vi "r_db_create.vi"(6 "ms timeout (0:default)":i32, 7 "db":string, 8 "error in (no error)":errorcluster, 11 "rethinkdb in":T1) -> (0 "error out":errorcluster, 1 "response":variant, 2 "db exists?":bool, 3 "rethinkdb out":T1)   [LabVIEW 2017, in "rethinkdb.lvlib"]
uses:
  rethinkdb.lvlib
  refnum.ctl
  ql2_term.ctl
  ql2_query.ctl
  ql2_term_to_id.vi
  ql2_query_to_id.vi
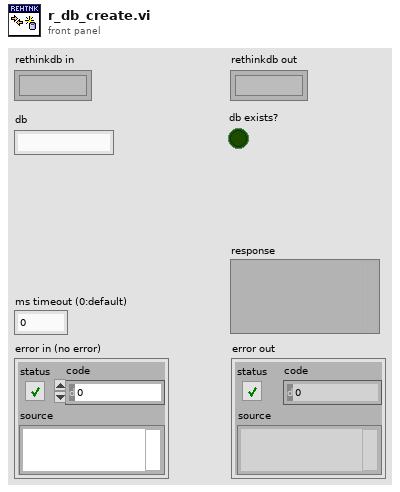
[diagram p1: front panel]
types:
  T1 = typedef "rethinkdb.lvlib/refnum.ctl" = refnum<k1>
  T2 = typedef "rethinkdb.lvlib/ql2_query.ctl" = enum8{"START", "CONTINUE", "STOP", "NOREPLY_WAIT", "SERVER_INFO", "invalid"}
  T3 = typedef "rethinkdb.lvlib/ql2_term.ctl" = enum8{"ADD", "AND", "APPEND", "APRIL", "ARGS", "ASC", "AUGUST", "AVG", "BETWEEN", "BETWEEN_DEPRECATED", "BINARY", "BIT_AND", "BIT_NOT", "BIT_OR", "BIT_SAL", "BIT_SAR", "BIT_XOR", "BRACKET", "BRANCH", "CEIL", "CHANGES", "CHANGE_AT", "CIRCLE", "COERCE_TO", "CONCAT_MAP", "CONFIG", "CONTAINS", "COUNT", "DATE", "DATUM", "DAY", "DAY_OF_WEEK", "DAY_OF_YEAR", "DB", "DB_CREATE", "DB_DROP", "DB_LIST", "DECEMBER", "DEFAULT", "DELETE", "DELETE_AT", "DESC", "DIFFERENCE", "DISTANCE", "DISTINCT", "DIV", "DOWNCASE", "DURING", "EPOCH_TIME", "EQ", "EQ_JOIN", "ERROR", "FEBRUARY", "FILL", "FILTER", "FLOOR", "FOLD", "FOR_EACH", "FRIDAY", "FUNC", "FUNCALL", "GE", "GEOJSON", "GET", "GET_ALL", "GET_FIELD", "GET_INTERSECTING", "GET_NEAREST", "GET_WRITE_HOOK", "GRANT", "GROUP", "GT", "HAS_FIELDS", "HOURS", "HTTP", "IMPLICIT_VAR", "INCLUDES", "INDEX_CREATE", "INDEX_DROP", "INDEX_LIST", "INDEX_RENAME", "INDEX_STATUS", "INDEX_WAIT", "INFO", "INNER_JOIN", "INSERT", "INSERT_AT", "INTERSECTS", "IN_TIMEZONE", "ISO8601", "IS_EMPTY", "JANUARY", "JAVASCRIPT", "JSON", "JULY", "JUNE", "KEYS", "LE", "LIMIT", "LINE", "LITERAL", "LT", "MAKE_ARRAY", "MAKE_OBJ", "MAP", "MARCH", "MATCH", "MAX", "MAXVAL", "MAY", "MERGE", "MIN", "MINUTES", "MINVAL", "MOD", "MONDAY", "MONTH", "MUL", "NE", "NOT", "NOVEMBER", "NOW", "NTH", "OBJECT", "OCTOBER", "OFFSETS_OF", "OR", "ORDER_BY", "OUTER_JOIN", "PLUCK", "POINT", "POLYGON", "POLYGON_SUB", "PREPEND", "RANDOM", "RANGE", "REBALANCE", "RECONFIGURE", "REDUCE", "REPLACE", "ROUND", "SAMPLE", "SATURDAY", "SECONDS", "SEPTEMBER", "SET_DIFFERENCE", "SET_INSERT", "SET_INTERSECTION", "SET_UNION", "SET_WRITE_HOOK", "SKIP", "SLICE", "SPLICE_AT", "SPLIT", "STATUS", "SUB", "SUM", "SUNDAY", "SYNC", "TABLE", "TABLE_CREATE", "TABLE_DROP", "TABLE_LIST", "THURSDAY", "TIME", "TIMEZONE", "TIME_OF_DAY", "TO_EPOCH_TIME", "TO_GEOJSON", "TO_ISO8601", "TO_JSON_STRING", "TUESDAY", "TYPE_OF", "UNGROUP", "UNION", "UPCASE", "UPDATE", "UUID", "VALUES", "VAR", "WAIT", "WEDNESDAY", "WITHOUT", "WITH_FIELDS", "YEAR", "ZIP", "invalid"}
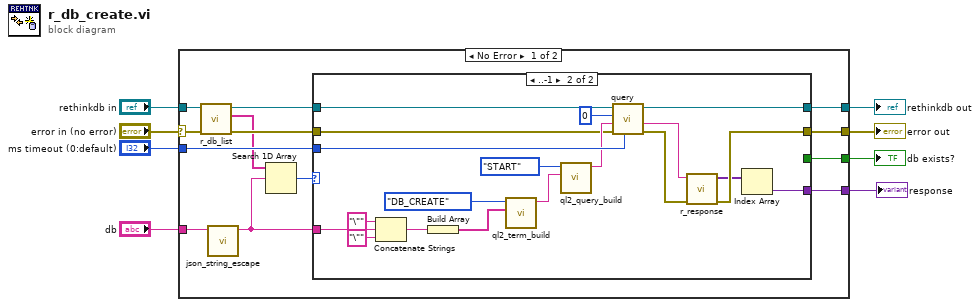
[diagram p0: block diagram]
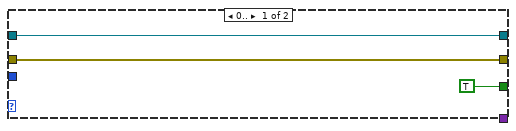
[diagram p2: hidden frame]
diagram:
  n1 = case shown="No Error" "error in (no error)" {
    selector: "error in (no error)" -> [w17 w45]
    tunnel: "rethinkdb in" -> [w15 w44]
    tunnel: [w21 w44] -> w6
    tunnel: "ms timeout (0:default)" -> [w20 _]
    tunnel: [w18 w45] -> w4
    tunnel: "db" -> [w19 _]
    tunnel: [w10 _] -> w2
    tunnel: [w9 _] -> w1
    frame No Error {
      n2 = call "r_db_list.vi"("error in (no error)"=w17, "rethinkdb in"=w15) -> ("error out"=w16:errorcluster, "db list"=w13:string[], "rethinkdb out"=w14:T1)  [unwired: 7 in]
      n3 = call "json_string_escape.vi"("string"=w19) -> ("escaped string"=w12:string)  [unwired: 10 in]
      n4 = Search 1D Array(1D array=w13, element=w12) -> (index of element=w11:i32)  [unwired: 1 in]
      n5 = case shown="..-1" w11 {
        tunnel: [w24 w43] -> w21
        tunnel: w20 -> [_ w42]
        tunnel: [w23 w30] -> w18
        tunnel: w16 -> [w23 w29]
        tunnel: w14 -> [w24 w28]
        tunnel: w12 -> [_ w27]
        tunnel: [TRUE _] -> w10
        tunnel: [_ w25] -> w9
        frame 0.. {
        }
        frame ..-1 {
          n6 = Concatenate Strings("\"" ("string"), w27, "\"" ("string")) -> (w32:string)
          n7 = Build Array(w32) -> (w31:string[])
          n8 = call "ql2_term_build.vi"("args"=w31, "term_type"=ql2_term."DB_CREATE") -> ("query"=w39:string)  [unwired: 9 in]
          n9 = call "ql2_query_build.vi"("query"=w39, "query_type"=ql2_query."START") -> ("query"=w40:string)  [unwired: 9 in]
          n10 = call "query.vi"("ms timeout (0:default)"=w42, "error in (no error)"=w29, "query"=w40, "token in (random)"=u64 0, "rethinkdb in"=w28) -> ("error out"=w38:errorcluster, "response"=w37:string, "rethinkdb out"=w43:T1)  [unwired: 3 in, 1 out]
          n11 = call "r_response.vi"("error in (no error)"=w38, "response"=w37) -> ("error out"=w30:errorcluster, "values"=w26:variant[])  [unwired: 8 in]
          n12 = Index Array(array=w26) -> (element=w25:variant)  [unwired: 1 in]
        }
      }
    }
    frame Error {
    }
  }
  "error out" <- w4
  "rethinkdb out" <- w6
  "db exists?" <- w2
  "response" <- w1
